vi "Actor Teardown.vi"(11 "Self Actor in":refnum<class "Self Actor.lvclass">) -> (2 "Teardown?":bool, 3 "Self Actor out":refnum<class "Self Actor.lvclass">)   [LabVIEW 2021, in "jettl.lvlib" / "Self Actor.lvclass"]
uses:
  Self Actor.lvclass
  C:/git/jettl/src/jettl/Actor/Actor.lvclass
  Self Actor.lvclass/Self Actor.ctl
  Self Actor State/Self Actor State.lvclass
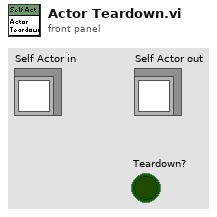
[diagram p1: front panel]
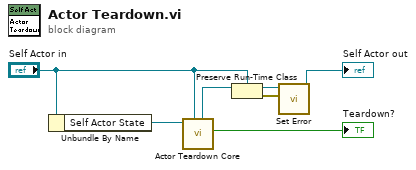
[diagram p0: block diagram]
diagram:
  n1 = Unbundle By Name("Self Actor in") -> ("Self Actor State"=w7:refnum<class "Self Actor State.lvclass">)
  n2 = call-dynamic "Actor Teardown Core.vi"("Actor in"="Self Actor in", "Self Actor State in"=w7) -> ("Teardown?"=→"Teardown?":bool, "Actor out"=w4:refnum<class "Actor.lvclass">)  [unwired: 8 in]
  n3 = Preserve Run-Time Class(object in=w4, 2:"Self Actor in") -> (object out=w3:refnum<class "Self Actor.lvclass">, error out=w1:errorcluster)  [unwired: 1 in]
  n4 = call-dynamic "Set Error.vi"("Error"=w1, "Self Actor in"=w3) -> ("Self Actor out"=→"Self Actor out":refnum<class "Self Actor.lvclass">)  [unwired: 9 in]
